vi "xiCam - GetLastImageParams.vi"(8 "error in (no error)":errorcluster, 11 "xiCam In":refnum<k24>) -> (0 "error out":errorcluster, 3 "xiCam Out":refnum<k24>, 4 "GetLastImageParams":refnum<k24>)   [LabVIEW 2016]
doc: "This function returns more detailed information about the last image in the ImgParams object"
uses:
  C:/Users/Ries Lab/Documents/Microscope Control from Sheng Account/Microscope-Control/Device Library/Cameras/Ximea/xiLIB_64bit/xiLIB/xiCamLib/API/x64/xiApi.NETX64.dll
  API/x64/xiApi.NETX64.dll
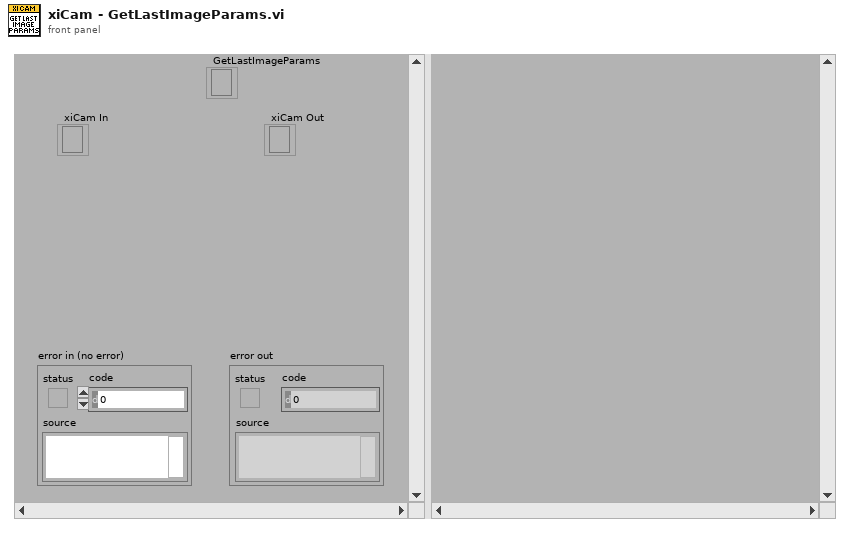
[diagram p1: front panel]
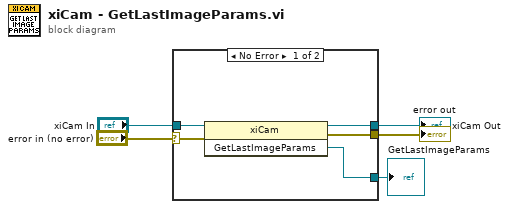
[diagram p0: block diagram]
diagram:
  n1 = case shown="No Error" "error in (no error)" {
    selector: "error in (no error)" -> [w8 w11]
    tunnel: "xiCam In" -> [w10 w12]
    tunnel: [w9 w12] -> w3
    tunnel: [w7 w11] -> w2
    tunnel: [w6 _] -> w1
    frame No Error {
      n2 = invoke class="xiCam" method="GetLastImageParams"(reference=w10, error in=w8) -> (reference out=w9:refnum<k24>, error out=w7:errorcluster, "GetLastImageParams"=w6:refnum<k24>)  [unwired: 1 in]
    }
    frame Error {
    }
  }
  "error out" <- w2
  "xiCam Out" <- w3
  "GetLastImageParams" <- w1
